vi "Mouse Acquire.vi"(8 "error in (no error)":errorcluster, 11 "UI_Top_Customer in":refnum<class "UI_Top_Customer.lvclass">) -> (0 "error out":errorcluster, 1 "button info":T1, 2 "axis info":T2, 3 "UI_Top_Customer out":refnum<class "UI_Top_Customer.lvclass">)   [LabVIEW 2021, in "UI_Top_Customer.lvclass"]
uses:
  UI_Top_Customer.lvclass
  C:/Program Files (x86)/National Instruments/LabVIEW 2021/user.lib/John_Lib/AbstractActorTemplate/AbstractActorTemplate/UIActorTop.lvclass
  UI_Top_Customer.lvclass/UI_Top_Customer.ctl
  <vilib>/Utility/inputDevices.llb/mouseAcquire.vi
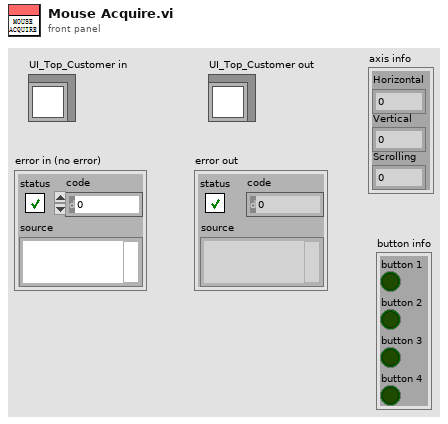
[diagram p1: front panel]
types:
  T1 = cluster{"button 1":bool, "button 2":bool, "button 3":bool, "button 4":bool}
  T2 = cluster{"Horizontal":i32, "Vertical":i32, "Scrolling":i32}
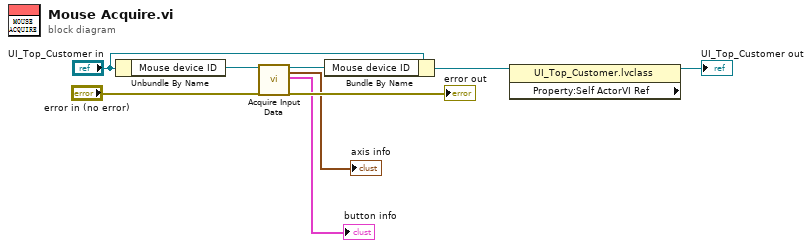
[diagram p0: block diagram]
diagram:
  n1 = Unbundle By Name("UI_Top_Customer in") -> ("Mouse device ID"=w8:refnum<k1>)
  n2 = call-poly <vilib>:"Acquire Input Data.vi"("device ID"=w8, "error in (no error)"="error in (no error)") -> ("device ID"=w6:refnum<k1>, "axis info"=→"axis info":T2, "button info"=→"button info":T1, "error out"=→"error out":errorcluster)  [unwired: 14 in]
  n3 = Bundle By Name(cluster="UI_Top_Customer in", "Mouse device ID"=w6) -> (w7:refnum<class "UI_Top_Customer.lvclass">)
  n4 = property class="UI_Top_Customer.lvclass" props=["Property:Self ActorVI Ref"](reference=w7) -> (reference out=→"UI_Top_Customer out":refnum<class "UI_Top_Customer.lvclass">)  [unwired: 1 in, 2 out]
